vi "Required Buffer Sizes.vi"(8 "error in (no error)":errorcluster, 11 "Framework Configuration in":refnum<class "Framework Configuration.lvclass">) -> (0 "error out":errorcluster, 1 "string size":u64 format="%d bytes", 2 "engine size":u64 format="%d bytes", 3 "Framework Configuration out":refnum<class "Framework Configuration.lvclass">)   [LabVIEW 2017, in "DSF Core.lvlib" / "Framework Configuration.lvclass"]
uses:
  Framework Configuration.lvclass
  Framework Configuration.lvclass/Framework Configuration.ctl
  Base/Plugin/Plugin Configuration.lvclass
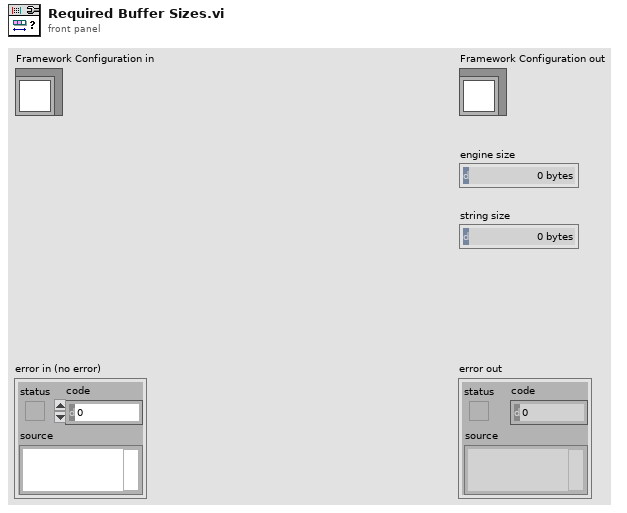
[diagram p1: front panel]
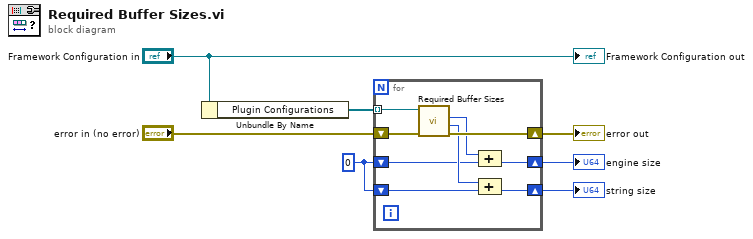
[diagram p0: block diagram]
diagram:
  w6 = u64 0 ("string size")
  n1 = Unbundle By Name("Framework Configuration in") -> ("Plugin Configurations"=w7:refnum<class "Plugin Configuration.lvclass">[])
  n2 = for {
    shift-right: [w16] -> w3
    shift-left: "error in (no error)" -> [w15]
    tunnel: w7 -> [w14] mode=indexing
    shift-right: [w10] -> w1
    shift-left: w6 -> [w11]
    shift-right: [w13] -> w2
    shift-left: w6 -> [w9]
    n3 = call-dynamic "Required Buffer Sizes.vi"("error in (no error)"=w15, "Plugin Configuration in"=w14) -> ("error out"=w16:errorcluster, "string size"=w12:u64, "engine size"=w8:u64)  [unwired: 6 in, 1 out]
    n4 = Compound Arithmetic op=ADD(w8, w11) -> (w10:u64)
    n5 = Compound Arithmetic op=ADD(w12, w9) -> (w13:u64)
  }
  "error out" <- w3
  "string size" <- w2
  "engine size" <- w1
  "Framework Configuration out" <- "Framework Configuration in"
